vi "set_range.vi"(8 "error in (no error)":errorcluster, 10 "VISA resource name in":refnum<visa-resource-name>, 11 "ComboBox in":refnum<vi>) -> (0 "error out":errorcluster, 3 "VISA Refnum out":refnum<visa-resource-name>)   [LabVIEW 2021]
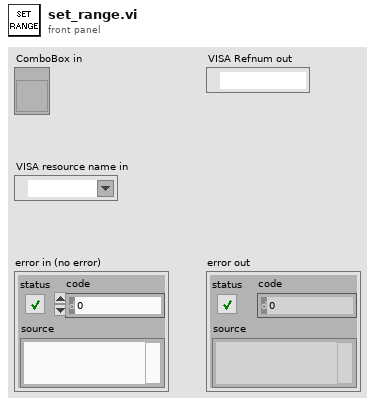
[diagram p1: front panel]
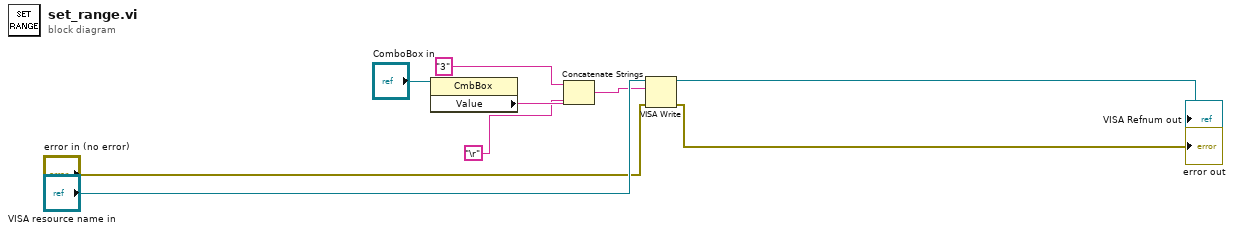
[diagram p0: block diagram]
diagram:
  n1 = property class="CmbBox"(reference="ComboBox in") -> ("Value"=w5:string)  [unwired: 1 in, 2 out]
  n2 = Concatenate Strings("3" ("string"), w5, "\r") -> (w3:string)
  n3 = VISA Write(VISA resource name="VISA resource name in", write buffer=w3, error in (no error)="error in (no error)") -> (VISA resource name out=→"VISA Refnum out":refnum<visa-resource-name>, error out=→"error out":errorcluster)  [unwired: 1 out]
